vi "Using Traverse.vi"() -> ()   [LabVIEW 2023]
doc: "This example shows how to use the Traverse for GObjects VI to search block diagrams and diagrams of structures for particular objects. The example also demonstrates how the recursive search functionality of Traverse for GObjects VI returns more information than the All Objects[] property."
uses:
  <vilib>/Utility/traverseref.llb/TRef TravTarget.ctl
  <vilib>/Utility/traverseref.llb/VI Scripting - Traverse.lvlib
panel:
  out "All Objects[]":string[][](table)
  out "Traverse For Loop Only":string[][](table)
  out "Traverse All":string[][](table)
  # "Overview: Demonstrates the use of the Traverse for GObjects VI to programmatically inspect the contents of a block diagram.\nInstructions:\n1. Open Test - Using Traverse.vi to see the block diagram being inspected.\n2. Run this VI. Observe the different object counts for the different ways (All Objects[], Traverse All, and Traverse For Loop Only) to inspect the diagram."
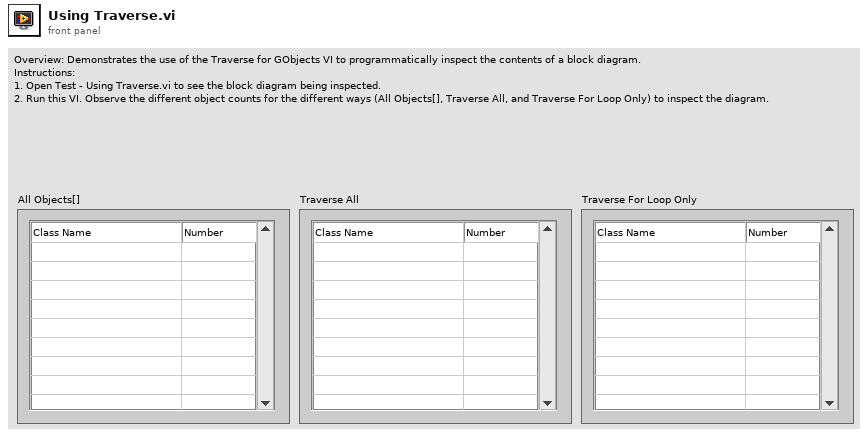
[diagram p1: front panel]
types:
  T1 = typedef "TRef TravTarget.ctl" = enum16{"FP", "BD", "Other"}
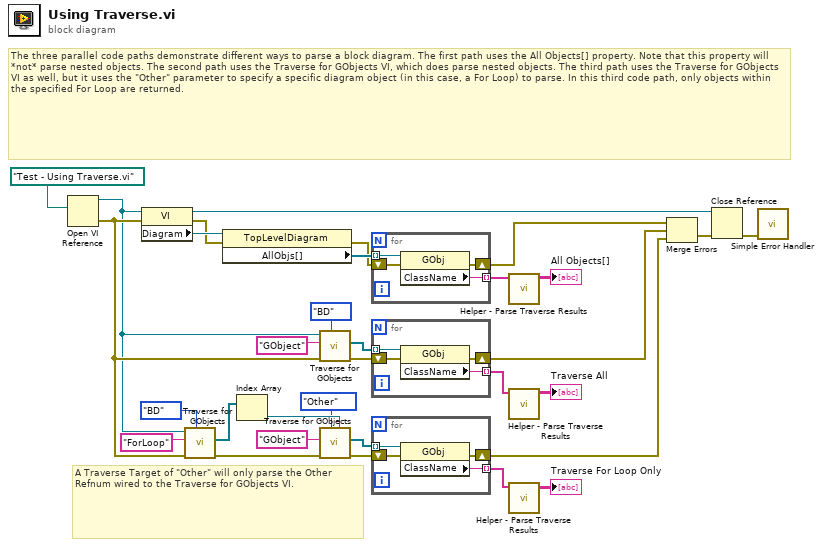
[diagram p0: block diagram]
diagram:
  # "A Traverse Target of \"Other\" will only parse the Other Refnum wired to the Traverse for GObjects VI."
  # "The three parallel code paths demonstrate different ways to parse a block diagram. The first path uses the All Objects[] property. Note that this property will *not* parse nested objects. The second path uses the Traverse for GObjects VI, which does parse nested objects. The third path uses the Traverse for GObjects VI as well, but it uses the \"Other\" parameter to specify a specific diagram object (in this case, a For Loop) to parse. In this third code path, only objects within the specified For Loop are returned."
  n1 = Open VI Reference(vi path=path "Test - Using Traverse.vi" ("Path to target VI")) -> (vi reference=w22:refnum<vi>, error out=w23:errorcluster)  [unwired: 5 in]
  n2 = property class="VI"(reference=w22, error in=w23) -> (reference out=w29:refnum<vi>, error out=w19:errorcluster, "Diagram"=w20:refnum<vi>)
  n3 = call <vilib>:"Traverse for GObjects.vi"("Traverse Target"=TRef_TravTarget."BD", "error in (no error)"=w23, "Class Name"="ForLoop", "VI Refnum"=w22) -> ("error out"=w25:errorcluster, "References"=w26:refnum<vi>[])  [unwired: 4 in, 2 out]
  n4 = property class="TopLevelDiagram"(reference=w20, error in=w19) -> (error out=w18:errorcluster, "AllObjs[]"=w21:refnum<vi>[])  [unwired: 1 out]
  n5 = Index Array(array=w26) -> (element=w27:refnum<vi>)  [unwired: 1 in]
  n6 = call <vilib>:"Traverse for GObjects.vi"("Traverse Target"=TRef_TravTarget."BD", "error in (no error)"=w23, "Class Name"="GObject", "VI Refnum"=w22) -> ("error out"=w11:errorcluster, "References"=w12:refnum<vi>[])  [unwired: 4 in, 2 out]
  n7 = call <vilib>:"Traverse for GObjects.vi"("Other Refnum"=w27, "Traverse Target"=TRef_TravTarget."Other", "error in (no error)"=w25, "Class Name"="GObject") -> ("error out"=w4:errorcluster, "References"=w3:refnum<vi>[])  [unwired: 4 in, 2 out]
  n8 = for {
    tunnel: w21 -> [w36] mode=indexing
    tunnel: [w35] -> w16 mode=indexing
    shift-right: [w33] -> w30
    shift-left: w18 -> [w34]
    n9 = property class="GObj"(reference=w36, error in=w34) -> (error out=w33:errorcluster, "ClassName"=w35:string)  [unwired: 1 out]
  }
  n10 = for {
    tunnel: w12 -> [w40] mode=indexing
    tunnel: [w39] -> w9 mode=indexing
    shift-right: [w37] -> w10
    shift-left: w11 -> [w38]
    n11 = property class="GObj"(reference=w40, error in=w38) -> (error out=w37:errorcluster, "ClassName"=w39:string)  [unwired: 1 out]
  }
  n12 = for {
    tunnel: w3 -> [w44] mode=indexing
    tunnel: [w43] -> w1 mode=indexing
    shift-right: [w41] -> w2
    shift-left: w4 -> [w42]
    n13 = property class="GObj"(reference=w44, error in=w42) -> (error out=w41:errorcluster, "ClassName"=w43:string)  [unwired: 1 out]
  }
  n14 = call "Helper - Parse Traverse Results.vi"("Traverse Results"=w16) -> ("Parsed Results"=→"All Objects[]":string[][])  [unwired: 10 in]
  n15 = call "Helper - Parse Traverse Results.vi"("Traverse Results"=w9) -> ("Parsed Results"=→"Traverse All":string[][])  [unwired: 10 in]
  n16 = call "Helper - Parse Traverse Results.vi"("Traverse Results"=w1) -> ("Parsed Results"=→"Traverse For Loop Only":string[][])  [unwired: 10 in]
  n17 = Merge Errors(w30, w10, w2) -> (w17:errorcluster)
  n18 = Close Reference(reference=w29, error in (no error)=w17) -> (error out=w31:errorcluster)
  n19 = call <vilib>:"Simple Error Handler.vi"("error in (no error)"=w31) -> ()  [unwired: 4 in, 5 out]
